vi "SUSLabPID.vi"() -> ()   [LabVIEW 2019]
uses:
  <vilib>/Utility/file.llb/Read Delimited Spreadsheet (DBL).vi
panel:
  in  "isAutomatic":bool=TRUE
  in  "isSimulated":bool=TRUE
  in  "isNoise":bool
  in  "Moc grza³ki":dbl(knob)=20.0 scale=0.0..100.0
  in  "Td":dbl=2.4
  in  "h":dbl=1.0 format="%#_13g"
  in  "Tzad":dbl=70.0
  in  "Ti":dbl=10.0
  in  "k":dbl=5.0
  out "ybez":dbl=81.78343971496386
  out "y":dbl=81.82654426687556
  in  "Thin":dbl=19.0
  in  "F":dbl=1.3
  in  "Delay":u32=10
  out "U":dbl=100.0
  in  "stop":bool
  out "Wykers":cluster{"Xwy":dbl, "Xwy":dbl, "Numeric":dbl}(graph)={"Xwy"=81.82654426687556, "Xwy"=30.360503637081145, "Numeric"=33.2}
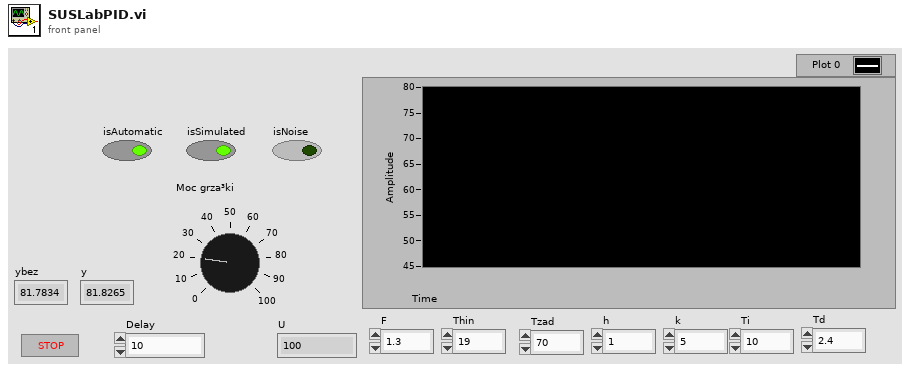
[diagram p1: front panel]
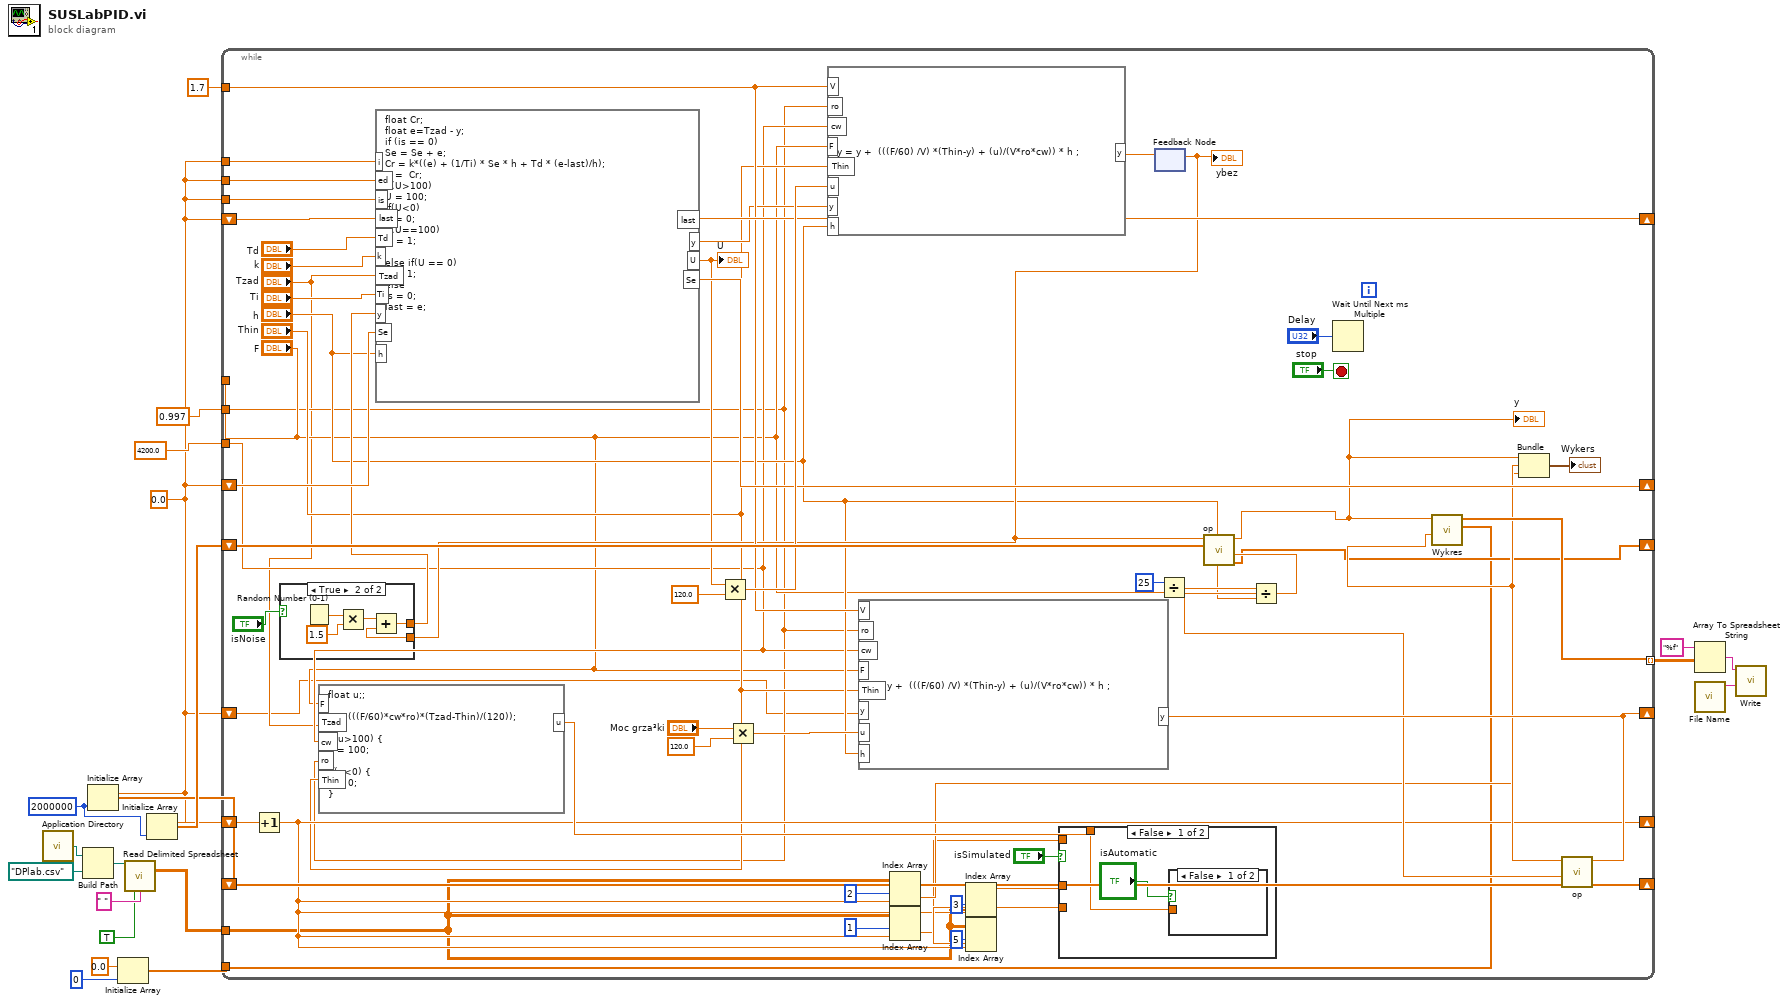
[diagram p0: block diagram]
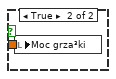
[diagram p2: hidden frame]
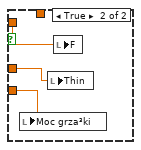
[diagram p3: hidden frame]
diagram:
  w3 = 2000000 ("dimension size")
  w2 = 0.0
  n1 = call <vilib>:"Application Directory.vi"() -> ("Application Directory"=w6:path)
  n2 = Build Path(base path=w6, name or relative path=path "DPlab.csv") -> (appended path=w4:path)
  n3 = Initialize Array(w2, w3) -> (w7:dbl[])
  n4 = Initialize Array(0.0 ("element"), 0 ("dimension size")) -> (w8:dbl[])
  n5 = call-poly <vilib>:"Read Delimited Spreadsheet.vi"("file path (dialog if empty)"=w4, "transpose? (F)"=TRUE, "delimiter (\\t)"=" " ("delimiter (\\t)")) -> ("all rows"=w1:dbl[][])  [unwired: 7 in, 5 out]
  n6 = Initialize Array(w2, w3) -> (w9:dbl[])
  n7 = while {
    tunnel: 1.7 ("V") -> [w56]
    tunnel: 0.997 ("ro") -> [w25]
    tunnel: 4200.0 ("cw") -> [w27]
    tunnel: [w58] -> w14 mode=indexing
    tunnel: w8 -> [w21]
    tunnel: ["F"] -> _
    shift-right: [w30] -> _
    shift-left: w9 -> [w75]
    shift-right: [w66] -> _
    shift-left: w2 -> [w67]
    shift-right: [w64] -> _
    shift-left: w2 -> [w32]
    shift-right: [w62] -> _
    shift-left: w2 -> [w23]
    shift-right: [w31] -> _
    shift-left: w7 -> [w59]
    shift-right: [w39] -> _
    shift-left: w2 -> [w48]
    tunnel: w2 -> [w36]
    tunnel: w2 -> [w35]
    tunnel: w2 -> [w33]
    tunnel: w1 -> [w22]
    stop <- "stop" stop-if-true
    n8 = Increment(x=w48) -> (x+1=w39:dbl)
    n9 = formula code="float u;;\n\nu = (((F/60)*cw*ro)*(Tzad-Thin)/(120));\n\nif(u>100) {\nu = 100;\n}\nif(u<0) {\nu = 0;\n}"("F"="F", "Tzad"="Tzad", "cw"=w27, "ro"=w25, "Thin"="Thin") -> ("u"=w45:dbl)
    n10 = Multiply(x="Moc grza³ki", y=120.0) -> (x*y=w51:dbl)
    n11 = formula code="y = y +  (((F/60) /V) *(Thin-y) + (u)/(V*ro*cw)) * h ;"("u"=w51, "y"=w23, "Thin"="Thin", "F"="F", "cw"=w27, "ro"=w25, "V"=w56, "h"="h") -> ("y"=w62:dbl)
    n12 = Index Array(array=w22, index (row)=2 ("disabled index (col)"), index (col)=w39) -> (element=w38:dbl)
    n13 = Index Array(array=w22, index (row)=1 ("disabled index (col)"), index (col)=w39) -> (element=w37:dbl)
    n14 = Index Array(array=w22, index (row)=3 ("disabled index (col)"), index (col)=w39) -> (element=w41:dbl)
    n15 = Index Array(array=w22, index (row)=5 ("disabled index (col)"), index (col)=w39) -> (element=w42:dbl)
    n16 = case shown="False" "isSimulated" {
      tunnel: w37 -> [_ w82]
      tunnel: w45 -> [w79 _]
      tunnel: w42 -> [_ w83]
      tunnel: w41 -> [_ w81]
      frame False {
        n17 = case shown="False" "isAutomatic" {
          tunnel: w79 -> [_ w80]
          frame False {
          }
          frame True {
            n18 = local write "Moc grza³ki"(w80) -> ()
          }
        }
      }
      frame True {
        n19 = local write "Moc grza³ki"(w83) -> ()
        n20 = local write "Thin"(w81) -> ()
        n21 = local write "F"(w82) -> ()
      }
    }
    n22 = feedback #1() -> (w53:dbl)  [unwired: 1 in]
    "ybez" <- w53
    n23 = case shown="True" "isNoise" {
      tunnel: w53 -> [w84 w87]
      tunnel: [w84 w85] -> w52
      frame False {
      }
      frame True {
        n24 = Random Number (0-1)() -> (number: 0 to 1=w89:dbl)
        n25 = Multiply(x=w89, y=1.5) -> (x*y=w86:dbl)
        n26 = Add(x=w86, y=w87) -> (x+y=w85:dbl)
      }
    }
    n27 = formula code="float Cr;\nfloat e=Tzad - y;\nif (is == 0) \nSe = Se + e;\nCr = k*((e) + (1/Ti) * Se * h + Td * (e-last)/h);\nU =  Cr;\nif(U>100) \nU = 100;\nif(U<0) \nU = 0;\nif(U==100) \nis = 1;\n\nelse if(U == 0) \nis = 1;\nelse \nis = 0;\nlast = e;"("k"="k", "Ti"="Ti", "Se"=w67, "y"=w52, "Tzad"="Tzad", "h"="h", "Td"="Td", "last"=w32, "is"=w33, "ed"=w36, "i"=w35) -> ("y"=w55:dbl, "U"=w34:dbl, "Se"=w66:dbl, "last"=w64:dbl)
    "U" <- w34
    n28 = Multiply(x=w34, y=120.0) -> (x*y=w70:dbl)
    n29 = formula code="y = y +  (((F/60) /V) *(Thin-y) + (u)/(V*ro*cw)) * h ;"("u"=w70, "y"=w55, "Thin"="Thin", "F"="F", "cw"=w27, "ro"=w25, "V"=w56, "h"="h") -> ("y"=w68:dbl)
    n30 = feedback-in #1(w68) -> ()
    n31 = Divide(x=25, y="F") -> (x/y=w61:dbl)
    n32 = Divide(x=w61, y="h") -> (x/y=w60:dbl)
    n33 = call "op.vi"("initialized array"=w75, "delay"=w60, "Xwe"=w53) -> ("s? t:f"=w30:dbl[], "Xwy"=w57:dbl)  [unwired: 7 in]
    "y" <- w57
    n34 = Wait Until Next ms Multiple(millisecond multiple="Delay") -> ()  [unwired: 1 out]
    n35 = call "op.vi"("initialized array"=w59, "delay"=w60, "Xwe"=w62) -> ("s? t:f"=w31:dbl[], "Xwy"=w49:dbl)  [unwired: 7 in]
    n36 = call "Wykres.vi"("new element/subarray"=w49, "initialized array"=w21, "Y"=w57) -> ("output array"=w58:dbl[])  [unwired: 8 in]
    n37 = Bundle("Xwy"=w57, "Xwy"=w49, "Numeric"=w38) -> (→"Wykers":cluster{"Xwy":dbl, "Xwy":dbl, "Numeric":dbl})  [unwired: 1 in]
  }
  n38 = Array To Spreadsheet String(array=w14, 3:"%f" ("format string")) -> (spreadsheet string=w12:string)  [unwired: 1 in]
  n39 = call "File Name.vi"() -> ("String"=w15:string)  [unwired: 11 in]
  n40 = call "Write.vi"("File Name"=w15, "text"=w12) -> ()  [unwired: 9 in, 1 out]
